vi "listen.vi"(8 "error in (no error)":errorcluster, 11 "SAL_Listener in":refnum<class "SAL_Listener.lvclass">) -> (0 "error out":errorcluster, 3 "SAL_Listener out":refnum<class "SAL_Listener.lvclass">)   [LabVIEW 2015, in "SAL_Listener.lvclass"]
uses:
  SAL_Listener.lvclass
  SAL_Listener.lvclass/SAL_Listener.ctl
  SALEvents/SAL_Events.lvclass/SAL_Events.ctl
  SALLV_dome/DataTypes/command_Park.ctl
  SALLV_dome/DataTypes/command_StopShutter.ctl
  SALLV_dome/DataTypes/command_OpenShutter.ctl
  SALLV_dome/DataTypes/command_CloseShutter.ctl
  SALLV_dome/DataTypes/command_start.ctl
  SALLV_dome/DataTypes/command_disable.ctl
  SALLV_dome/DataTypes/command_enable.ctl
  SALLV_dome/DataTypes/command_exitControl.ctl
  SALLV_dome/DataTypes/command_standby.ctl
  SALLV_dome/DataTypes/command_stop.ctl
  SALLV_dome/DataTypes/command_Move.ctl
  SALLV_dome/DataTypes/command_Crawl.ctl
  SALLV_dome/DataTypes/command_SetLouvers.ctl
  SALEvents/SAL_Events.lvclass
  SALLV_dome/SALLV_dome.lvlib
  SALLV_domeADB/SALLV_domeADB.lvlib
panel:
  out "stopIsTrue":bool
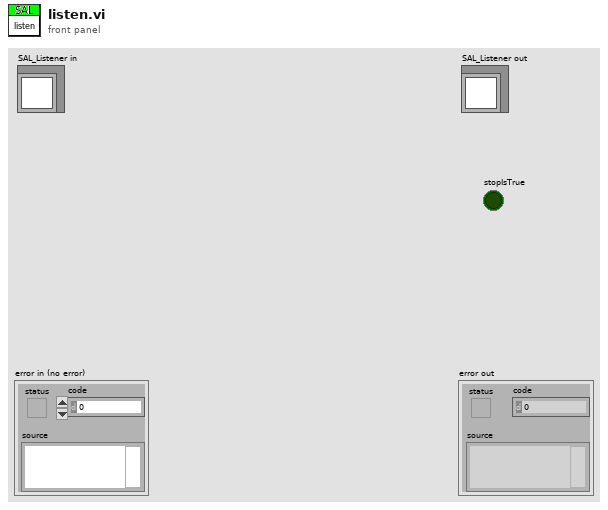
[diagram p1: front panel]
types:
  T1 = typedef "sharedEvents.ctl" = cluster{"stopApp":refnum<user-event>}
  T2 = typedef "commandsEvents.ctl" = cluster{"start":refnum<user-event>, "disable":refnum<user-event>, "enable":refnum<user-event>, "exitControl":refnum<user-event>, "standby":refnum<user-event>, "stop":refnum<user-event>, "move":refnum<user-event>, "crawl":refnum<user-event>, "setLouvers":refnum<user-event>, "Park":refnum<user-event>, "StopShutter":refnum<user-event>, "OpenShutter":refnum<user-event>, "CloseShutter":refnum<user-event>}
  T3 = cluster{"Event Registration Refnum":refnum<event-registration>, "SALEventEventRef":refnum<event-registration>, "SALTelemetryEventRef":refnum<event-registration>}
  T4 = typedef "SALLV_dome.lvlib/command_Park.ctl" = cluster{"state":bool}
  T5 = typedef "SALLV_dome.lvlib/command_StopShutter.ctl" = cluster{"state":bool}
  T6 = typedef "SALLV_dome.lvlib/command_OpenShutter.ctl" = cluster{"state":bool}
  T7 = typedef "SALLV_dome.lvlib/command_CloseShutter.ctl" = cluster{"state":bool}
  T8 = typedef "SALLV_dome.lvlib/command_start.ctl" = cluster{"configuration":string}
  T9 = typedef "SALLV_dome.lvlib/command_disable.ctl" = cluster{"state":bool}
  T10 = typedef "SALLV_dome.lvlib/command_enable.ctl" = cluster{"state":bool}
  T11 = typedef "SALLV_dome.lvlib/command_exitControl.ctl" = cluster{"state":bool}
  T12 = typedef "SALLV_dome.lvlib/command_standby.ctl" = cluster{"state":bool}
  T13 = typedef "SALLV_dome.lvlib/command_stop.ctl" = cluster{"state":bool}
  T14 = typedef "SALLV_dome.lvlib/command_Move.ctl" = cluster{"azimuth":dbl, "elevation":dbl}
  T15 = typedef "SALLV_dome.lvlib/command_Crawl.ctl" = cluster{"azPosition":dbl, "elPosition":dbl, "demandTime":i32}
  T16 = typedef "SALLV_dome.lvlib/command_SetLouvers.ctl" = cluster{"position[34]":i32[]}
  T17 = typedef "eventsEvents.ctl" = cluster{"AppliedSettingsMatchStart":refnum<user-event>, "ErrorCode":refnum<user-event>, "SettingVersions":refnum<user-event>, "StateChanged":refnum<user-event>, "SummaryState":refnum<user-event>}
  T18 = typedef "telemetryEvents.ctl" = cluster{"ADBstatus":refnum<user-event>}
  T19 = typedef "SALLV_dome.lvlib/logevent_AppliedSettingsMatchStart.ctl" = cluster{"appliedSettingsMatchStartIsTrue":bool, "priority":i32}
  T20 = typedef "SALLV_dome.lvlib/logevent_ErrorCode.ctl" = cluster{"errorCode":i32, "priority":i32}
  T21 = typedef "SALLV_dome.lvlib/logevent_SettingVersions.ctl" = cluster{"recommendedSettingVersion":string, "priority":i32}
  T22 = typedef "SALLV_dome.lvlib/logevent_StateChanged.ctl" = cluster{"newState":i32, "priority":i32}
  T23 = typedef "SALLV_dome.lvlib/logevent_SummaryState.ctl" = cluster{"SummaryStateValue":i32, "priority":i32}
  T24 = typedef "SALLV_domeADB.lvlib/status.ctl" = cluster{"position_error":sgl, "position_actual":sgl, "position_cmd":sgl, "drive_torque_actual[5]":sgl[], "drive_torque_error[5]":sgl[], "drive_torque_cmd[5]":sgl[], "drive_current_actual[5]":sgl[], "drive_temp_actual[5]":sgl[], "encoder_head_raw[5]":sgl[], "encoder_head_calibrated[5]":sgl[], "resolver_raw[5]":sgl[], "resolver_calibrated[5]":sgl[]}
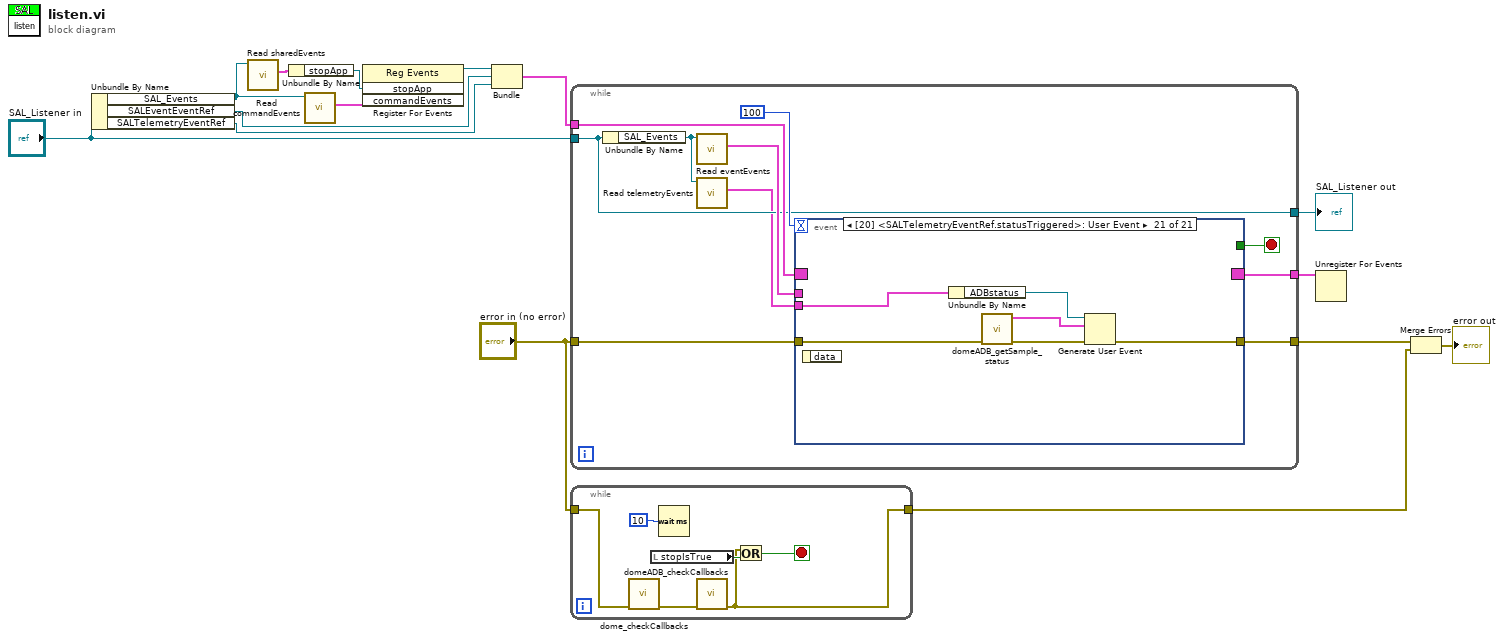
[diagram p0: block diagram]
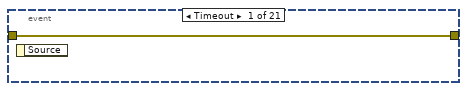
[diagram p2: hidden frame]
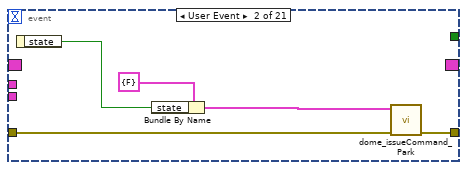
[diagram p3: hidden frame]
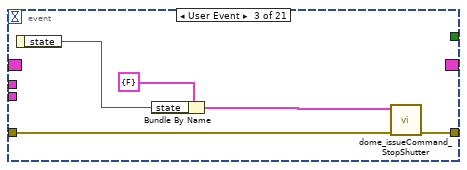
[diagram p4: hidden frame]
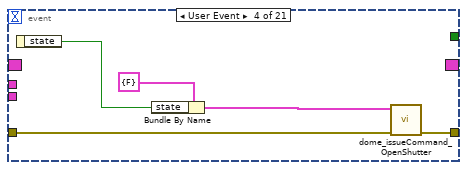
[diagram p5: hidden frame]
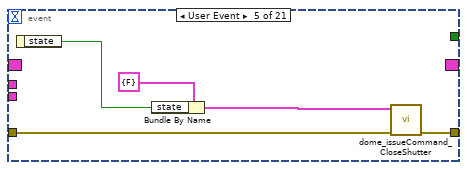
[diagram p6: hidden frame]
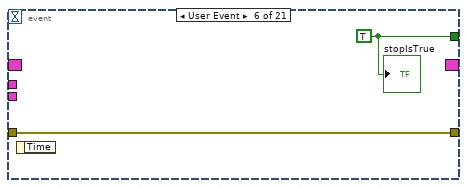
[diagram p7: hidden frame]
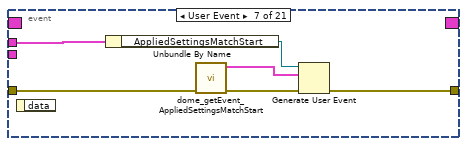
[diagram p8: hidden frame]
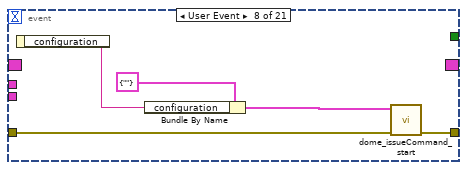
[diagram p9: hidden frame]
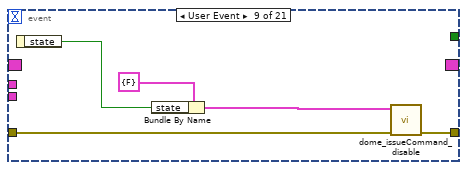
[diagram p10: hidden frame]
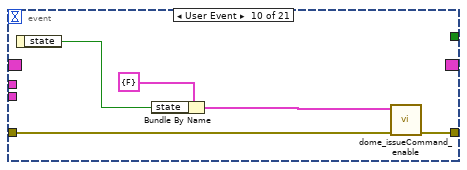
[diagram p11: hidden frame]
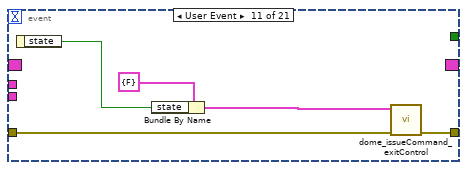
[diagram p12: hidden frame]
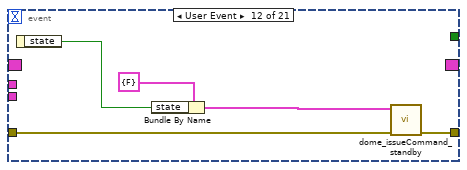
[diagram p13: hidden frame]
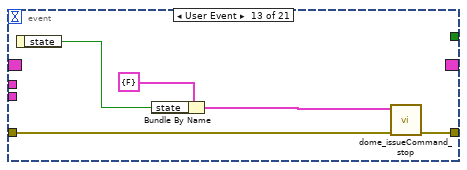
[diagram p14: hidden frame]
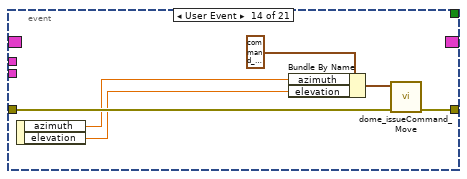
[diagram p15: hidden frame]
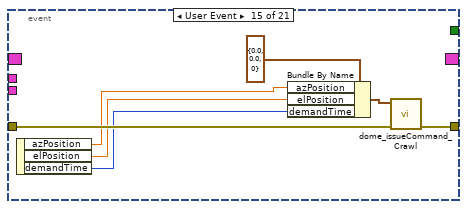
[diagram p16: hidden frame]
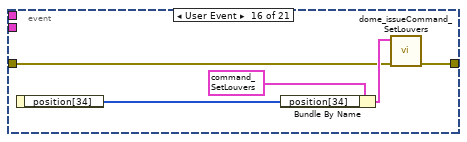
[diagram p17: hidden frame]
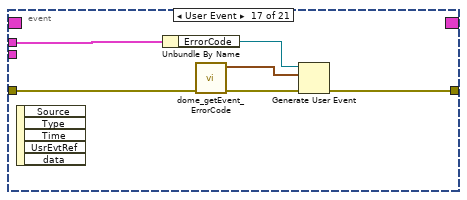
[diagram p18: hidden frame]
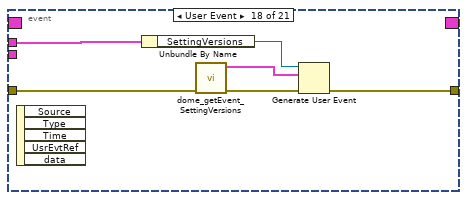
[diagram p19: hidden frame]
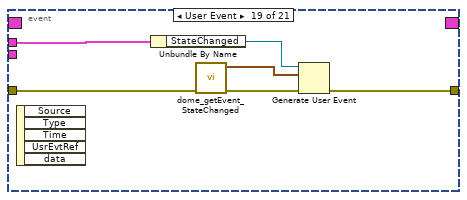
[diagram p20: hidden frame]
diagram:
  n1 = Unbundle By Name("SAL_Listener in") -> ("SAL_Events"=w7:refnum<class "SAL_Events.lvclass">, "SALEventEventRef"=w15:refnum<event-registration>, "SALTelemetryEventRef"=w1:refnum<event-registration>)
  n2 = call "Read sharedEvents.vi"("SAL_Events in"=w7) -> ("sharedEvents"=w10:T1)  [unwired: 8 in, 2 out]
  n3 = Unbundle By Name(w10) -> ("stopApp"=w9:refnum<user-event>)
  n4 = call "Read commandEvents.vi"("SAL_Events in"=w7) -> ("commandEvents"=w6:T2)  [unwired: 8 in, 2 out]
  n5 = register-events(w9, w6) -> (reference out=w8:refnum<event-registration>)  [unwired: 2 in, 1 out]
  n6 = Bundle("Event Registration Refnum"=w8, "SALEventEventRef"=w15, "SALTelemetryEventRef"=w1) -> (w14:T3)  [unwired: 1 in]
  n7 = while {
    tunnel: w14 -> [w25]
    tunnel: [w24] -> w13
    tunnel: "SAL_Listener in" -> [w18]
    tunnel: [w18] -> w11
    tunnel: [w21] -> w4
    tunnel: "error in (no error)" -> [w20]
    stop <- w23 stop-if-true
    n8 = Unbundle By Name(w18) -> ("SAL_Events"=w17:refnum<class "SAL_Events.lvclass">)
    n9 = call "Read eventEvents.vi"("SAL_Events in"=w17) -> ("eventEvents"=w22:T17)  [unwired: 8 in, 2 out]
    n10 = call "Read telemetryEvents.vi"("SAL_Events in"=w17) -> ("telemetryEvents"=w16:T18)  [unwired: 8 in, 2 out]
    n11 = event shown="[20] <SALTelemetryEventRef.statusTriggered>: User Event" {
      selector: w25 -> [_ _ _ _ _ _ _ _ _ _ _ _ _ _ _ _ _ _ _ _ _]
      dyn-events: [_ _ _ _ _ _ _ _ _ _ _ _ _ _ _ _ _ _ _ _ _] -> w24
      timeout: 100 -> [_ _ _ _ _ _ _ _ _ _ _ _ _ _ _ _ _ _ _ _ _]
      tunnel: [_ _ _ _ _ w47 _ _ _ _ _ _ _ _ _ _ _ _ _ _ _] -> w23
      tunnel: w22 -> [_ _ _ _ _ _ w53 _ _ _ _ _ _ _ _ _ w104 w110 w116 w122 _]
      tunnel: [w26 w27 w32 w37 w45 w48 w49 w58 w61 w67 w71 w76 w81 w88 w94 w98 w103 w109 w115 w121 w129] -> w21
      tunnel: w20 -> [w26 w28 w33 w38 w46 w48 w54 w59 w62 w66 w72 w77 w82 w87 w95 w99 w108 w114 w120 w126 w132]
      tunnel: w16 -> [_ _ _ _ _ _ _ _ _ _ _ _ _ _ _ _ _ _ _ _ w131]
      event Timeout {
        n12 = event-data() -> ()  [unwired: 1 in, 1 out]
      }
      event User Event {
        n13 = event-data() -> ("state"=w30:bool)  [unwired: 1 in]
        n14 = Bundle By Name(cluster=T4 {"state"=FALSE} ("command_Park_Ctl"), "state"=w30) -> (w29:T4)
        n15 = call "dome_issueCommand_Park.vi"("error in (no error)"=w28, "command_Park_Ctl"=w29) -> ("error out"=w27:errorcluster)  [unwired: 7 in, 2 out]
      }
      event User Event {
        n16 = event-data() -> ("state"=w35:bool)  [unwired: 1 in]
        n17 = Bundle By Name(cluster=T5 {"state"=FALSE} ("command_StopShutter_Ctl"), "state"=w35) -> (w34:T5)
        n18 = call "dome_issueCommand_StopShutter.vi"("error in (no error)"=w33, "command_StopShutter_Ctl"=w34) -> ("error out"=w32:errorcluster)  [unwired: 7 in, 2 out]
      }
      event User Event {
        n19 = event-data() -> ("state"=w39:bool)  [unwired: 1 in]
        n20 = Bundle By Name(cluster=T6 {"state"=FALSE} ("command_OpenShutter_Ctl"), "state"=w39) -> (w40:T6)
        n21 = call "dome_issueCommand_OpenShutter.vi"("error in (no error)"=w38, "command_OpenShutter_Ctl"=w40) -> ("error out"=w37:errorcluster)  [unwired: 7 in, 2 out]
      }
      event User Event {
        n22 = event-data() -> ("state"=w42:bool)  [unwired: 1 in]
        n23 = Bundle By Name(cluster=T7 {"state"=FALSE} ("command_CloseShutter_Ctl"), "state"=w42) -> (w43:T7)
        n24 = call "dome_issueCommand_CloseShutter.vi"("error in (no error)"=w46, "command_CloseShutter_Ctl"=w43) -> ("error out"=w45:errorcluster)  [unwired: 7 in, 2 out]
      }
      event User Event {
        w47 = TRUE
        n25 = event-data() -> ()  [unwired: 1 in, 1 out]
        "stopIsTrue" <- w47
      }
      event User Event {
        n26 = event-data() -> ()  [unwired: 1 in, 1 out]
        n27 = Unbundle By Name(w53) -> ("AppliedSettingsMatchStart"=w52:refnum<user-event>)
        n28 = call "dome_getEvent_AppliedSettingsMatchStart.vi"("error in (no error)"=w54) -> ("error out"=w50:errorcluster, "logevent_AppliedSettingsMatchStart_Ctl out"=w51:T19)  [unwired: 8 in, 1 out]
        n29 = Generate User Event(user event=w52, event data cluster=w51, error in=w50) -> (error out=w49:errorcluster)  [unwired: 1 in, 1 out]
      }
      event User Event {
        n30 = event-data() -> ("configuration"=w55:string)  [unwired: 1 in]
        n31 = Bundle By Name(cluster=T8 {"configuration"=""} ("command_start_Ctl"), "configuration"=w55) -> (w57:T8)
        n32 = call "dome_issueCommand_start.vi"("error in (no error)"=w59, "command_start_Ctl"=w57) -> ("error out"=w58:errorcluster)  [unwired: 7 in, 2 out]
      }
      event User Event {
        n33 = event-data() -> ("state"=w60:bool)  [unwired: 1 in]
        n34 = Bundle By Name(cluster=T9 {"state"=FALSE} ("command_disable_Ctl"), "state"=w60) -> (w63:T9)
        n35 = call "dome_issueCommand_disable.vi"("error in (no error)"=w62, "command_disable_Ctl"=w63) -> ("error out"=w61:errorcluster)  [unwired: 7 in, 2 out]
      }
      event User Event {
        n36 = event-data() -> ("state"=w65:bool)  [unwired: 1 in]
        n37 = Bundle By Name(cluster=T10 {"state"=FALSE} ("command_enable_Ctl"), "state"=w65) -> (w68:T10)
        n38 = call "dome_issueCommand_enable.vi"("error in (no error)"=w66, "command_enable_Ctl"=w68) -> ("error out"=w67:errorcluster)  [unwired: 7 in, 2 out]
      }
      event User Event {
        n39 = event-data() -> ("state"=w70:bool)  [unwired: 1 in]
        n40 = Bundle By Name(cluster=T11 {"state"=FALSE} ("command_exitControl_Ctl"), "state"=w70) -> (w73:T11)
        n41 = call "dome_issueCommand_exitControl.vi"("error in (no error)"=w72, "command_exitControl_Ctl"=w73) -> ("error out"=w71:errorcluster)  [unwired: 7 in, 2 out]
      }
      event User Event {
        n42 = event-data() -> ("state"=w75:bool)  [unwired: 1 in]
        n43 = Bundle By Name(cluster=T12 {"state"=FALSE} ("command_standby_Ctl"), "state"=w75) -> (w78:T12)
        n44 = call "dome_issueCommand_standby.vi"("error in (no error)"=w77, "command_standby_Ctl"=w78) -> ("error out"=w76:errorcluster)  [unwired: 7 in, 2 out]
      }
      event User Event {
        n45 = event-data() -> ("state"=w83:bool)  [unwired: 1 in]
        n46 = Bundle By Name(cluster=T13 {"state"=FALSE} ("command_stop_Ctl"), "state"=w83) -> (w80:T13)
        n47 = call "dome_issueCommand_stop.vi"("error in (no error)"=w82, "command_stop_Ctl"=w80) -> ("error out"=w81:errorcluster)  [unwired: 7 in, 2 out]
      }
      event User Event {
        n48 = event-data() -> ("azimuth"=w86:dbl, "elevation"=w85:dbl)  [unwired: 1 in]
        n49 = Bundle By Name(cluster=T14 {"azimuth"=0.0, "elevation"=0.0} ("command_Move_Ctl"), "azimuth"=w86, "elevation"=w85) -> (w89:T14)
        n50 = call "dome_issueCommand_Move.vi"("error in (no error)"=w87, "command_Move_Ctl"=w89) -> ("error out"=w88:errorcluster)  [unwired: 7 in, 2 out]
      }
      event User Event {
        n51 = event-data() -> ("azPosition"=w93:dbl, "elPosition"=w92:dbl, "demandTime"=w91:i32)  [unwired: 1 in]
        n52 = Bundle By Name(cluster=T15 {"azPosition"=0.0, "elPosition"=0.0, "demandTime"=0} ("command_Crawl_Ctl"), "azPosition"=w93, "elPosition"=w92, "demandTime"=w91) -> (w96:T15)
        n53 = call "dome_issueCommand_Crawl.vi"("error in (no error)"=w95, "command_Crawl_Ctl"=w96) -> ("error out"=w94:errorcluster)  [unwired: 7 in, 2 out]
      }
      event User Event {
        n54 = event-data() -> ("position[34]"=w101:i32[])  [unwired: 1 in]
        n55 = Bundle By Name(cluster=T16 {"position[34]"=[0, 0, 0, 0, 0, 0, 0, 0, 0, 0, 0, 0, 0, 0, 0, 0, 0, 0, 0, 0, 0, 0, 0, 0, 0, 0, 0, 0, 0, 0, 0, 0, 0, 0]} ("command_SetLouvers_Ctl"), "position[34]"=w101) -> (w100:T16)
        n56 = call "dome_issueCommand_SetLouvers.vi"("error in (no error)"=w99, "command_SetLouvers_Ctl"=w100) -> ("error out"=w98:errorcluster)  [unwired: 7 in, 2 out]
      }
      event User Event {
        n57 = event-data() -> ()  [unwired: 1 in, 5 out]
        n58 = Unbundle By Name(w104) -> ("ErrorCode"=w107:refnum<user-event>)
        n59 = call "dome_getEvent_ErrorCode.vi"("error in (no error)"=w108) -> ("error out"=w105:errorcluster, "logevent_ErrorCode_Ctl out"=w106:T20)  [unwired: 8 in, 1 out]
        n60 = Generate User Event(user event=w107, event data cluster=w106, error in=w105) -> (error out=w103:errorcluster)  [unwired: 1 in, 1 out]
      }
      event User Event {
        n61 = event-data() -> ()  [unwired: 1 in, 5 out]
        n62 = Unbundle By Name(w110) -> ("SettingVersions"=w113:refnum<user-event>)
        n63 = call "dome_getEvent_SettingVersions.vi"("error in (no error)"=w114) -> ("error out"=w111:errorcluster, "logevent_SettingVersions_Ctl out"=w112:T21)  [unwired: 8 in, 1 out]
        n64 = Generate User Event(user event=w113, event data cluster=w112, error in=w111) -> (error out=w109:errorcluster)  [unwired: 1 in, 1 out]
      }
      event User Event {
        n65 = event-data() -> ()  [unwired: 1 in, 5 out]
        n66 = Unbundle By Name(w116) -> ("StateChanged"=w119:refnum<user-event>)
        n67 = call "dome_getEvent_StateChanged.vi"("error in (no error)"=w120) -> ("error out"=w118:errorcluster, "logevent_StateChanged_Ctl out"=w117:T22)  [unwired: 8 in, 1 out]
        n68 = Generate User Event(user event=w119, event data cluster=w117, error in=w118) -> (error out=w115:errorcluster)  [unwired: 1 in, 1 out]
      }
      event User Event {
        n69 = event-data() -> ()  [unwired: 1 in, 1 out]
        n70 = Unbundle By Name(w122) -> ("SummaryState"=w125:refnum<user-event>)
        n71 = call "dome_getEvent_SummaryState.vi"("error in (no error)"=w126) -> ("error out"=w124:errorcluster, "logevent_SummaryState_Ctl out"=w123:T23)  [unwired: 8 in, 1 out]
        n72 = Generate User Event(user event=w125, event data cluster=w123, error in=w124) -> (error out=w121:errorcluster)  [unwired: 1 in, 1 out]
      }
      event User Event {
        n73 = event-data() -> ()  [unwired: 1 in, 1 out]
        n74 = Unbundle By Name(w131) -> ("ADBstatus"=w128:refnum<user-event>)
        n75 = call "domeADB_getSample_status.vi"("error in (no error)"=w132) -> ("error out"=w130:errorcluster, "status_Ctl out"=w127:T24)  [unwired: 8 in, 1 out]
        n76 = Generate User Event(user event=w128, event data cluster=w127, error in=w130) -> (error out=w129:errorcluster)  [unwired: 1 in, 1 out]
      }
    }
  }
  "SAL_Listener out" <- w11
  n77 = while {
    tunnel: "error in (no error)" -> [w136]
    tunnel: [w133] -> w2
    stop <- w137 stop-if-true
    n78 = call "dome_checkCallbacks.vi"("error in (no error)"=w136) -> ("error out"=w134:errorcluster)  [unwired: 10 in]
    n79 = local read "stopIsTrue"() -> (w138:bool)
    n80 = Wait (ms)(milliseconds to wait=u32 10) -> ()  [unwired: 1 out]
    n81 = call "domeADB_checkCallbacks.vi"("error in (no error)"=w134) -> ("error out"=w133:errorcluster)  [unwired: 10 in]
    n82 = Or(x=w133, y=w138) -> (x .or. y?=w137:bool)
  }
  n83 = Unregister For Events(event registration refnum=w13) -> ()  [unwired: 1 in, 1 out]
  n84 = Merge Errors(w4, w2) -> (→"error out":errorcluster)
